vi "Mean Phase.vi"(7 "modulus":enum16{"2pi", "1", "360"}(ring), 11 "phase":dbl[](array[numeric])) -> (2 "R":dbl, 3 "mean phase":dbl)   [LabVIEW 2012]
uses:
  <vilib>/Analysis/baseanly.llb/Mean (DBL).vi
  <vilib>/Analysis/NI_AALBase.lvlib
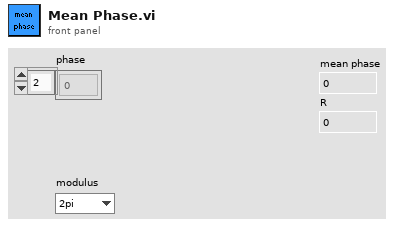
[diagram p1: front panel]
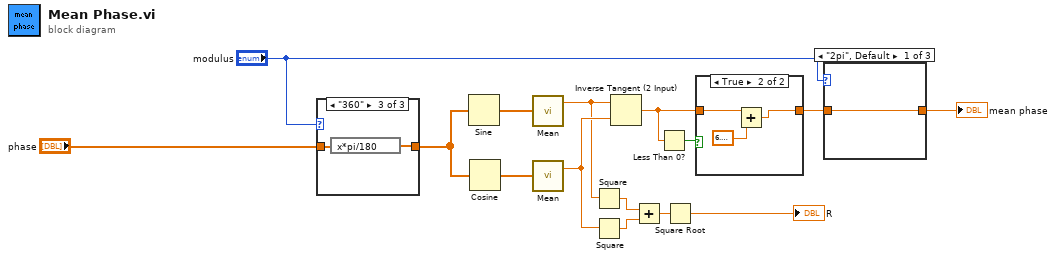
[diagram p0: block diagram]
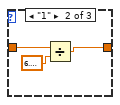
[diagram p3: hidden frame]
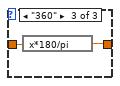
[diagram p4: hidden frame]
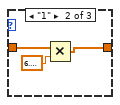
[diagram p6: hidden frame]
diagram:
  n1 = case shown="\"360\"" "modulus" {
    tunnel: "phase" -> [w16 w19 w21]
    tunnel: [w16 w17 w20] -> w8
    frame "2pi", Default {
    }
    frame "1" {
      n2 = Multiply(x=w19, y=6.283185307179586) -> (x*y=w17:dbl[])
    }
    frame "360" {
      n3 = expression code="x*pi/180"(w21) -> (w20:dbl[])
    }
  }
  n4 = Sine(x=w8) -> (sin(x)=w15:dbl[])
  n5 = Cosine(x=w8) -> (cos(x)=w14:dbl[])
  n6 = call-poly <vilib>:"Mean.vi"("X"=w15) -> ("mean"=w12:dbl)  [unwired: 1 out]
  n7 = call-poly <vilib>:"Mean.vi"("X"=w14) -> ("mean"=w13:dbl)  [unwired: 1 out]
  n8 = Square(x=w12) -> (x^2=w10:dbl)
  n9 = Square(x=w13) -> (x^2=w11:dbl)
  n10 = Inverse Tangent (2 Input)(1:w13, 2:w12) -> (0:w2:dbl)
  n11 = Add(x=w10, y=w11) -> (x+y=w9:dbl)
  n12 = Less Than 0?(x=w2) -> (x < 0?=w3:bool)
  n13 = Square Root(x=w9) -> (sqrt(x)=→"R":dbl)
  n14 = case shown="True" w3 {
    tunnel: w2 -> [w22 w25]
    tunnel: [w22 w23] -> w1
    frame False {
    }
    frame True {
      n15 = Add(x=w25, y=6.283185307179586) -> (x+y=w23:dbl)
    }
  }
  n16 = case shown="\"2pi\", Default" "modulus" {
    tunnel: w1 -> [w26 w29 w31]
    tunnel: [w26 w27 w30] -> w6
    frame "2pi", Default {
    }
    frame "1" {
      n17 = Divide(x=w29, y=6.283185307179586) -> (x/y=w27:dbl)
    }
    frame "360" {
      n18 = expression code="x*180/pi"(w31) -> (w30:dbl)
    }
  }
  "mean phase" <- w6
